vi "FTW-DevUtil-FrontPanelCleanup.vi"() -> ()   [LabVIEW 2014]
panel:
  out "error out":errorcluster
  in  "Path":path
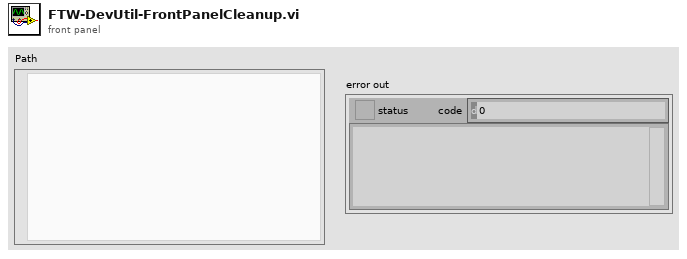
[diagram p1: front panel]
types:
  T1 = cluster{"Left":i16, "Top":i16, "Right":i16, "Bottom":i16}
  T2 = enum16{"No Scaling", "Scale All Objects", "Scale Single Object"}
  T3 = enum16{"Always On", "Always Off", "Off While Running"}
  T4 = typedef "LVRectTypeDef.ctl" = cluster{"Left":i16, "Top":i16, "Right":i16, "Bottom":i16}
  T5 = enum32{"invalid VI type", "Standard VI", "Control VI", "Global VI", "Polymorphic VI", "Configuration VI", "SubSystem", "Facade VI", "Method VI", "Statechart Diagram VI"}
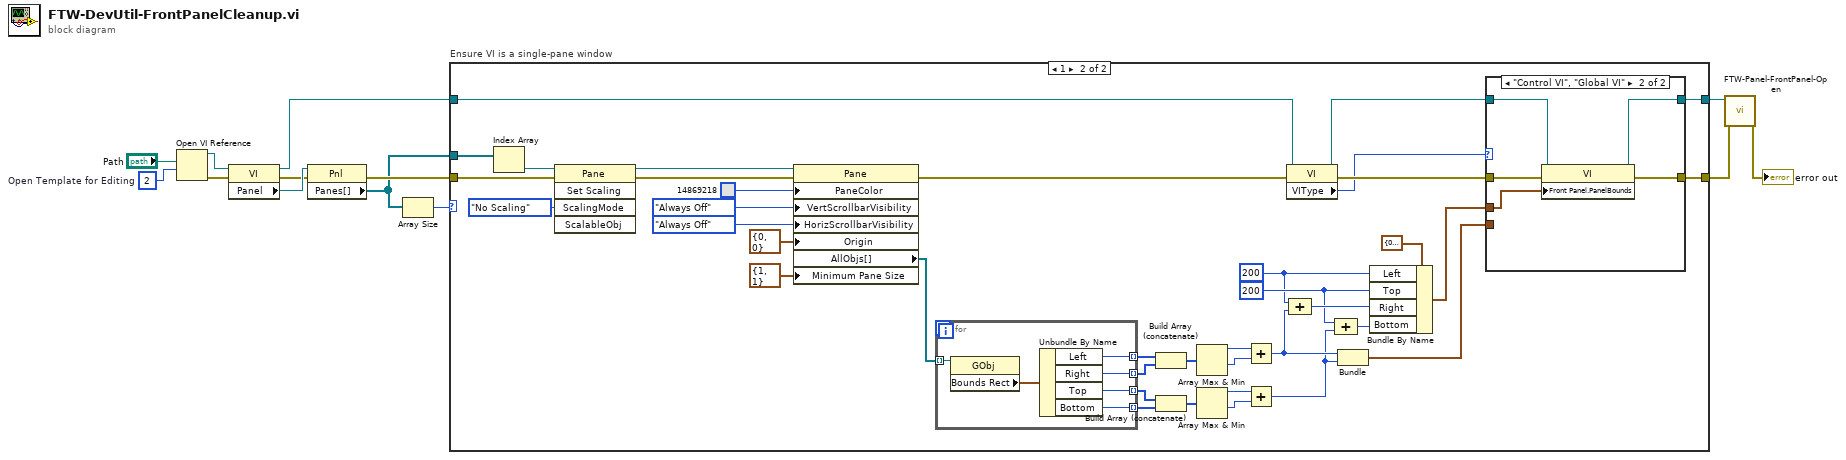
[diagram p0: block diagram]
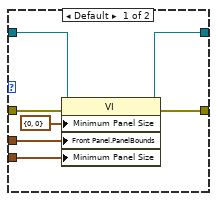
[diagram p3: hidden frame]
diagram:
  w4 = 2  # Open Template for Editing
  n1 = Open VI Reference(vi path="Path", options=w4) -> (vi reference=w12:refnum<vi>, error out=w10:errorcluster)  [unwired: 4 in]
  n2 = property class="VI"(reference=w12, error in=w10) -> (reference out=w3:refnum<vi>, error out=w9:errorcluster, "Panel"=w11:refnum<vi>)
  n3 = property class="Pnl"(reference=w11, error in=w9) -> (error out=w8:errorcluster, "Panes[]"=w7:refnum<vi>[])  [unwired: 1 out]
  n4 = Array Size(array=w7) -> (size(s)=w6:i32)
  n5 = case "Ensure VI is a single-pane window" shown="1" w6 {
    tunnel: w8 -> [w15 w36]
    tunnel: [w15 w42] -> w5
    tunnel: w7 -> [_ w43]
    tunnel: w3 -> [w14 w17]
    tunnel: [w14 w27] -> w2
    frame Default {
    }
    frame 1 {
      w24 = i16 200 ("Left")
      w23 = i16 200 ("Left")
      n6 = Index Array(array=w43) -> (element=w37:refnum<vi>)  [unwired: 1 in]
      n7 = invoke class="Pane" method="Set Scaling"(reference=w37, error in=w36, "ScalingMode"=T2."No Scaling" ("Scaling Mode")) -> (reference out=w34:refnum<vi>, error out=w35:errorcluster)  [unwired: 2 in, 3 out]
      n8 = property class="Pane"(reference=w34, error in=w35, "PaneColor"=u32 14869218, "VertScrollbarVisibility"=T3."Always Off" ("Vertical Scrollbar Visibility"), "HorizScrollbarVisibility"=T3."Always Off" ("Vertical Scrollbar Visibility"), "Origin"=cluster{"Horizontal":i16, "Vertical":i16} {"Horizontal"=0, "Vertical"=0}, "Minimum Pane Size"=cluster{"Horizontal":i16, "Vertical":i16} {"Horizontal"=1, "Vertical"=1}) -> (error out=w20:errorcluster, "AllObjs[]"=w50:refnum<vi>[])  [unwired: 1 out]
      n9 = for {
        tunnel: w50 -> [w71] mode=indexing
        tunnel: [w70] -> w49 mode=indexing
        tunnel: [w69] -> w48 mode=indexing
        tunnel: [w68] -> w46 mode=indexing
        tunnel: [w67] -> w45 mode=indexing
        n10 = property class="GObj"(reference=w71) -> ("Bounds Rect"=w66:T4)  [unwired: 1 in, 2 out]
        n11 = Unbundle By Name(w66) -> ("Left"=w70:i16, "Right"=w69:i16, "Top"=w68:i16, "Bottom"=w67:i16)
      }
      n12 = Build Array (concatenate)(w49, w48) -> (w47:i16[])
      n13 = Build Array (concatenate)(w46, w45) -> (w44:i16[])
      n14 = Array Max & Min(array=w47) -> (max value=w31:i16, min value=w30:i16)  [unwired: 2 out]
      n15 = Array Max & Min(array=w44) -> (max value=w33:i16, min value=w32:i16)  [unwired: 2 out]
      n16 = Add(x=w31, y=w30) -> (x+y=w29:i16)
      n17 = Add(x=w33, y=w32) -> (x+y=w28:i16)
      n18 = property class="VI"(reference=w17, error in=w20) -> (reference out=w16:refnum<vi>, error out=w19:errorcluster, "VIType"=w18:T5)
      n19 = Compound Arithmetic op=ADD(w23, w29) -> (w26:i16)
      n20 = Compound Arithmetic op=ADD(w24, w28) -> (w25:i16)
      n21 = Bundle(w29, w28) -> (w21:cluster{i16, i16})  [unwired: 1 in]
      n22 = Bundle By Name(cluster=T1 {"Left"=0, "Top"=0, "Right"=0, "Bottom"=0} ("Front Panel Window:Panel Bounds"), "Left"=w23, "Top"=w24, "Right"=w26, "Bottom"=w25) -> (w41:T1)
      n23 = case shown="\"Control VI\", \"Global VI\"" w18 {
        tunnel: [w60 w65] -> w42
        tunnel: w41 -> [w59 w64]
        tunnel: [w58 w63] -> w27
        tunnel: w16 -> [w57 w62]
        tunnel: w21 -> [w56 _]
        tunnel: w19 -> [w55 w61]
        frame Default {
          n24 = property class="VI"(reference=w57, error in=w55, "Minimum Panel Size"=cluster{"Horizontal":i16, "Vertical":i16} {"Horizontal"=0, "Vertical"=0} ("Front Panel Window:Minimum Size"), "Front Panel.PanelBounds"=w59, "Minimum Panel Size"=w56) -> (reference out=w58:refnum<vi>, error out=w60:errorcluster)
        }
        frame "Control VI", "Global VI" {
          n25 = property class="VI"(reference=w62, error in=w61, "Front Panel.PanelBounds"=w64) -> (reference out=w63:refnum<vi>, error out=w65:errorcluster)
        }
      }
    }
  }
  n26 = call "FTW-Panel-FrontPanel-Open.vi"("error in"=w5, "VI Ref"=w2) -> ("error out"=→"error out":errorcluster)  [unwired: 8 in, 1 out]
